vi "Laser Daq - SubVI.vi"(11 "Array":bool[](array[boolean])=[FALSE, FALSE, FALSE]) -> ()   [LabVIEW 2014]
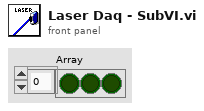
[diagram p1: front panel]
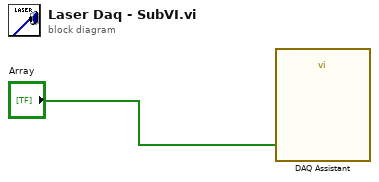
[diagram p0: block diagram]
diagram:
  n1 = call "DAQ Assistant"("data"="Array") -> ()  [unwired: 17 in, 2 out]
